vi "tag bus tags to cvt tags.vi"(11 "TB Tags":refnum<class "tag descriptor.lvclass">[](array[class])) -> (3 "CVT Tags":T1[](array[typedef]))   [LabVIEW 2013, in "CVT Engine Configuration.lvclass"]
uses:
  CVT Engine Configuration.lvclass
  <vilib>/NI/Current Value Table/Type Defs/Single Tag.ctl
  <vilib>/NI/Current Value Table/Type Defs/Data Types.ctl
  <vilib>/NI/Tag Bus/tag/tag descriptor.lvclass
  <vilib>/NI/Tag Bus/tag/tag descriptor.lvclass/tag descriptor.ctl
  <vilib>/NI/Current Value Table/Current Value Table.lvlib
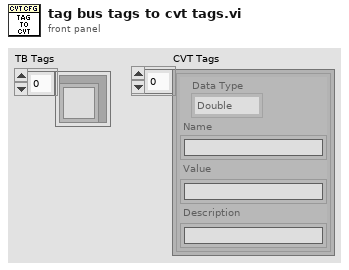
[diagram p1: front panel]
types:
  T1 = typedef "Current Value Table.lvlib/Single Tag.ctl" = cluster{"Data Type":T2, "Name":string, "Value":string, "Description":string}
  T2 = typedef "Current Value Table.lvlib/Data Types.ctl" = enum16{"Double", "Single", "I64", "I32", "I16", "I8", "U64", "U32", "U16", "U8", "String", "Boolean", "Array of U8", "Array of U16", "Array of U32", "Array of U64", "Array of I64", "Array of I32", "Array of I16", "Array of I8", "Array of Double", "Array of Single", "Array of Boolean", "Array of String"}
  T3 = typedef "tag bus.lvlib/tag descriptor.lvclass/Data Type.ctl" = enum16{"Double", "Single", "I64", "I32", "I16", "I8", "U64", "U32", "U16", "U8", "Boolean", "String", "Array of Double", "Array of Single", "Array of I64", "Array of I32", "Array of I16", "Array of I8", "Array of U64", "Array of U32", "Array of U16", "Array of U8", "Array of Boolean", "Array of String"}
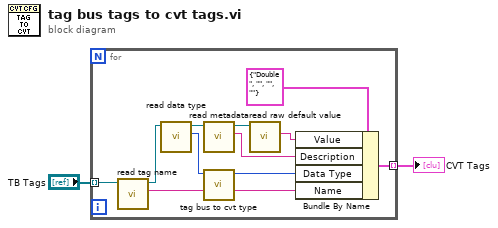
[diagram p0: block diagram]
diagram:
  n1 = for {
    tunnel: "TB Tags" -> [w13] mode=indexing
    tunnel: [w8] -> w1 mode=indexing
    n2 = call <vilib>:"read tag name.vi"("system tag in"=w13) -> ("name"=w3:string, "system tag out"=w12:refnum<class "tag descriptor.lvclass">)  [unwired: 8 in, 1 out]
    n3 = call <vilib>:"read data type.vi"("system tag in"=w12) -> ("data type"=w7:T3, "system tag out"=w10:refnum<class "tag descriptor.lvclass">)  [unwired: 8 in, 1 out]
    n4 = call <vilib>:"read metadata.vi"("system tag in"=w10) -> ("metadata"=w5:string, "system tag out"=w11:refnum<class "tag descriptor.lvclass">)  [unwired: 8 in, 1 out]
    n5 = call "tag bus to cvt type.vi"("Data Type"=w7) -> ("cvt type"=w4:T2)  [unwired: 10 in]
    n6 = call <vilib>:"read raw default value.vi"("system tag in"=w11) -> ("raw default"=w6:string)  [unwired: 8 in, 2 out]
    n7 = Bundle By Name(cluster=T1 {"Data Type"=enum."Double", "Name"="", "Value"="", "Description"=""} ("Tag"), "Value"=w6, "Description"=w5, "Data Type"=w4, "Name"=w3) -> (w8:T1)
  }
  "CVT Tags" <- w1
